vi "genData.vi"() -> ()   [LabVIEW 2020]
uses:
  <vilib>/Analysis/baseanly.llb/Mean (DBL).vi
  <vilib>/Analysis/NI_AALBase.lvlib
panel:
  out "property values":variant[](array[variant])
  out "property names":string[](array[string])
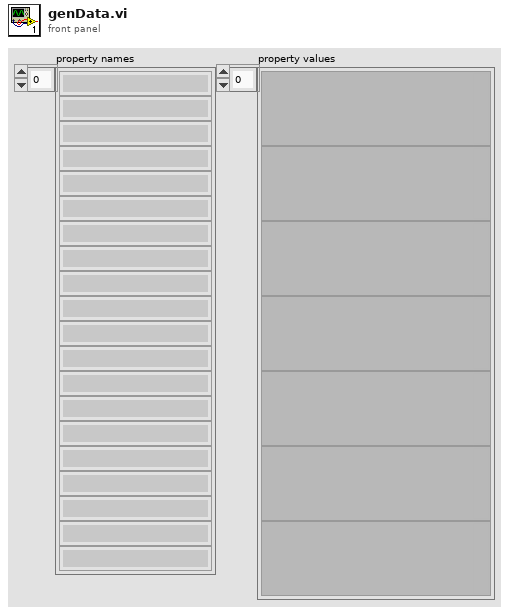
[diagram p1: front panel]
types:
  T1 = enum16{"open", "open or create", "create or replace", "create", "open (read-only)"}
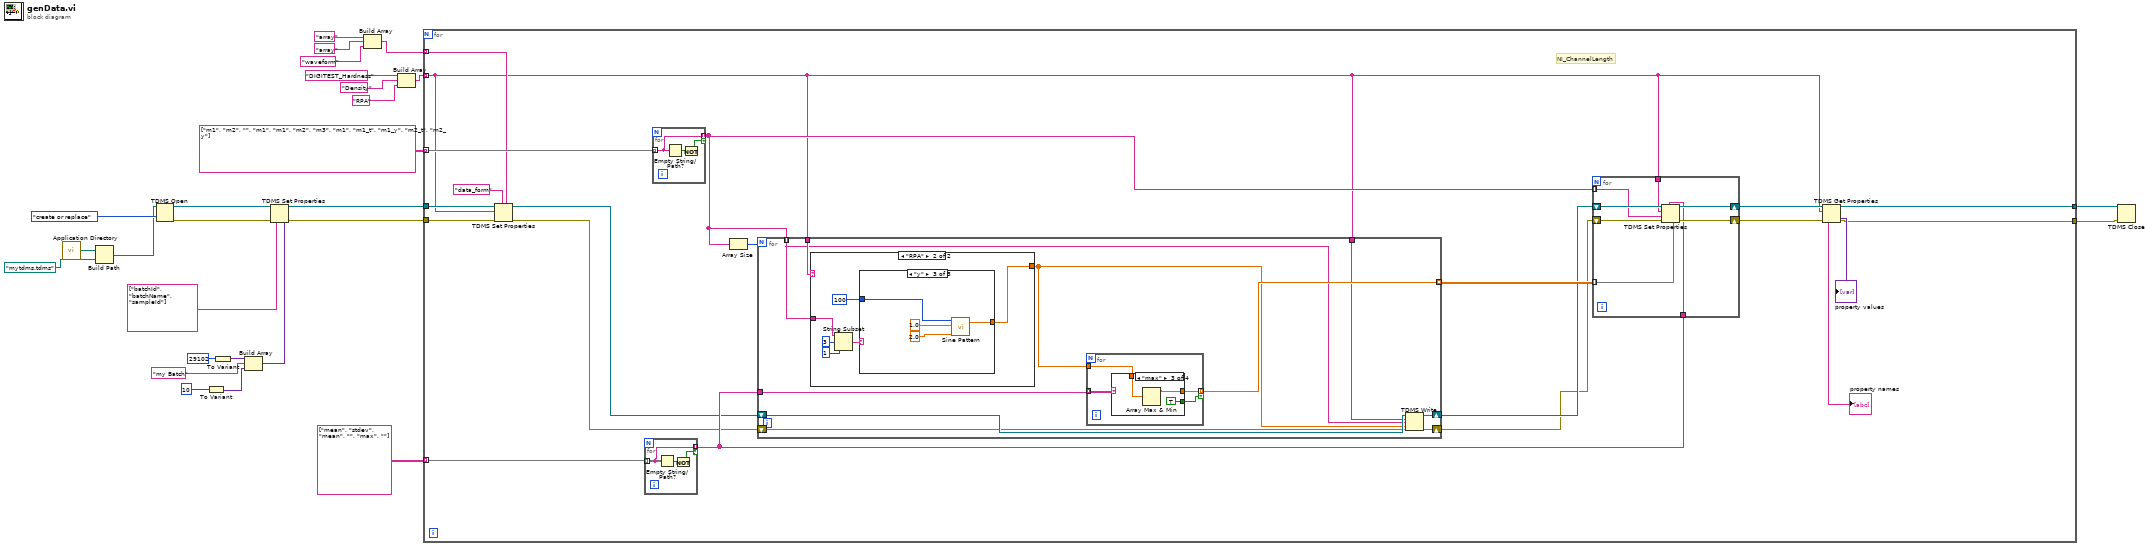
[diagram p0: block diagram]
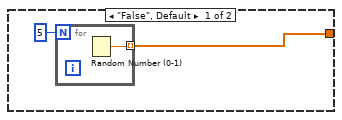
[diagram p2: hidden frame]
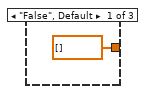
[diagram p3: hidden frame]
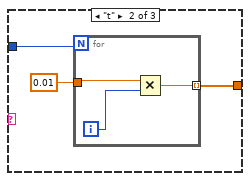
[diagram p4: hidden frame]
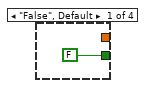
[diagram p5: hidden frame]
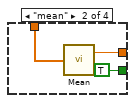
[diagram p6: hidden frame]
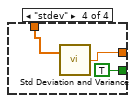
[diagram p7: hidden frame]
diagram:
  n1 = call <vilib>:"Application Directory.vi"() -> ("Application Directory"=w18:path)
  n2 = Build Path(base path=w18, name or relative path=path "mytdms.tdms" ("file path")) -> (appended path=w16:path)
  n3 = TDMS Open(10:T1."create or replace" ("operation (0:open)"), 11:w16) -> (0:w14:errorcluster, 3:w15:refnum<k34>)  [unwired: 5 in]
  n4 = To Variant(anything=10) -> (Variant=w5:variant)
  n5 = To Variant(anything=29102) -> (Variant=w9:variant)
  n6 = Build Array(w9, "my Batch", w5) -> (w8:variant[])
  n7 = TDMS Set Properties(5:w8, 7:string[] ["batchId", "batchName", "sampleId"] ("property names"), 8:w14, 11:w15) -> (0:w12:errorcluster, 3:w13:refnum<k34>)  [unwired: 2 in, 2 out]
  n8 = Build Array("array" ("group name in (Untitled)"), "array" ("group name in (Untitled)"), "waveform" ("group name in (Untitled)")) -> (w1:string[])
  n9 = Build Array("DIGITEST_Hardness" ("group name in (Untitled)"), "Density" ("group name in (Untitled)"), "RPA" ("group name in (Untitled)")) -> (w24:string[])
  n10 = for {
    tunnel: w13 -> [w34]
    tunnel: w24 -> [w28] mode=indexing
    tunnel: string[][] [["m1", "m2", "", "m1"], ["m1", "m2", "m3", "m1"], ["m1_t", "m1_y", "m2_t", "m2_y"]] -> [w43] mode=indexing
    tunnel: string[][] [["mean", "stdev"], ["mean", ""], ["max", ""]] ("property names") -> [w41] mode=indexing
    tunnel: w12 -> [w33]
    tunnel: [w39] -> w21
    tunnel: [w38] -> w20
    tunnel: w1 -> [w30] mode=indexing
    # "NI_ChannelLength"
    n11 = TDMS Set Properties(5:w30, 7:"data_form" ("property names"), 8:w33, 10:w28, 11:w34) -> (0:w32:errorcluster, 3:w31:refnum<k34>)  [unwired: 1 in, 2 out]
    n12 = for {
      tunnel: w41 -> [w51] mode=indexing
      tunnel: [w51] -> w40 mode=indexing if=w49
      n13 = Empty String/Path?(string/path=w51) -> (empty?=w50:bool)
      n14 = Not(x=w50) -> (.not. x?=w49:bool)
    }
    n15 = for {
      tunnel: w43 -> [w54] mode=indexing
      tunnel: [w54] -> w37 mode=indexing if=w52
      n16 = Empty String/Path?(string/path=w54) -> (empty?=w53:bool)
      n17 = Not(x=w53) -> (.not. x?=w52:bool)
    }
    n18 = Array Size(array=w37) -> (size(s)=w42:i32)
    n19 = for {
      N: w42 -> [_]
      tunnel: [w71] -> w44 mode=indexing
      tunnel: w40 -> [w72]
      tunnel: w28 -> [w69]
      tunnel: w37 -> [w63] mode=indexing
      shift-right: [w68] -> w36
      shift-left: w31 -> [w70]
      shift-right: [w67] -> w35
      shift-left: w32 -> [w66]
      tunnel: w28 -> [w65]
      n20 = case shown="\"RPA\"" w65 {
        tunnel: [w73 w76] -> w64
        tunnel: w63 -> [_ w81]
        frame "False", Default {
          n21 = for {
            N: 5 -> [_]
            tunnel: [w75] -> w73 mode=indexing
            n22 = Random Number (0-1)() -> (number: 0 to 1=w75:dbl)
          }
        }
        frame "RPA" {
          n23 = String Subset(string=w81, offset (0)=3, length (rest)=1 ("length (rest)")) -> (substring=w78:string)
          n24 = case shown="\"y\"" w78 {
            tunnel: 100 -> [_ w85 w91]
            tunnel: [dbl[] [] ("Sinusoidal Pattern") w83 w89] -> w76
            frame "False", Default {
            }
            frame "t" {
              n25 = for {
                N: w85 -> [_]
                tunnel: 0.01 -> [w88]
                tunnel: [w86] -> w83 mode=indexing
                i -> [w87]
                n26 = Multiply(x=w88, y=w87) -> (x*y=w86:dbl)
              }
            }
            frame "y" {
              n27 = call <vilib>:"Sine Pattern.vi"("cycles"=2.0, "amplitude"=1.0, "samples"=w91) -> ("Sinusoidal Pattern"=w89:dbl[])  [unwired: 1 in, 1 out]
            }
          }
        }
      }
      n28 = for {
        tunnel: w72 -> [w96] mode=indexing
        tunnel: w64 -> [w95]
        tunnel: [w94] -> w71 mode=indexing if=w93
        n29 = case shown="\"max\"" w96 {
          tunnel: w95 -> [_ w100 w102 w106]
          tunnel: [_ w99 w101 w105] -> w94
          tunnel: [FALSE TRUE TRUE TRUE] -> w93
          frame "False", Default {
          }
          frame "mean" {
            n30 = call-poly <vilib>:"Mean.vi"("X"=w100) -> ("mean"=w99:dbl)  [unwired: 1 out]
          }
          frame "max" {
            n31 = Array Max & Min(array=w102) -> (max value=w101:dbl)  [unwired: 3 out]
          }
          frame "stdev" {
            n32 = call <vilib>:"Std Deviation and Variance.vi"("X"=w106) -> ("standard deviation"=w105:dbl)  [unwired: 1 in, 2 out]
          }
        }
      }
      n33 = TDMS Write(0:w70, 5:w69, 7:w63, 9:w64, 11:w66) -> (4:w68:refnum<k34>, 15:w67:errorcluster)  [unwired: 1 in, 2 out]
    }
    n34 = for {
      tunnel: w28 -> [w60]
      shift-right: [w58] -> w45
      shift-left: w36 -> [w62]
      shift-right: [w59] -> w46
      shift-left: w35 -> [w61]
      tunnel: w37 -> [w57] mode=indexing
      tunnel: w44 -> [w56] mode=indexing
      tunnel: w40 -> [w55]
      n35 = TDMS Set Properties(5:w56, 7:w55, 8:w61, 9:w57, 10:w60, 11:w62) -> (0:w59:errorcluster, 3:w58:refnum<k34>)  [unwired: 2 out]
    }
    n36 = TDMS Get Properties(8:w46, 10:w28, 11:w45) -> (0:w39:errorcluster, 3:w38:refnum<k34>, 4:→"property values":variant[], 6:→"property names":string[])  [unwired: 3 in, 2 out]
  }
  n37 = TDMS Close(8:w21, 11:w20) -> ()  [unwired: 2 out]
